vi "Event handler-Restart.vi"(11 "Queue in":refnum<queue>) -> (0 "error out":errorcluster)   [LabVIEW 2013]
uses:
  Queue/Message Queue/Typedefs/Message Cluster.ctl
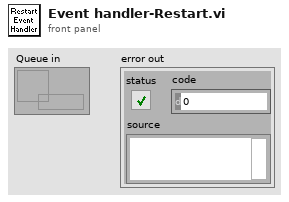
[diagram p1: front panel]
types:
  T1 = enum32{"Invalid", "Standard", "Closed", "Hidden", "Minimized", "Maximized"}
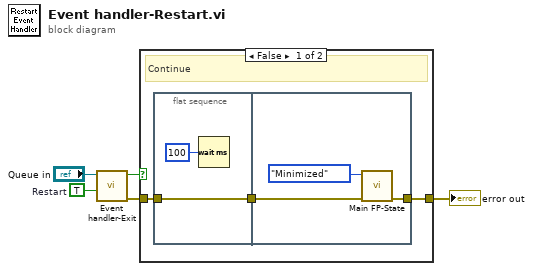
[diagram p0: block diagram]
diagram:
  w5 = TRUE  # Restart
  n1 = call "Event handler-Exit.vi"("Restart (F)"=w5, "UI queue"="Queue in") -> ("error out"=w1:errorcluster, "Cancelled"=w4:bool)  [unwired: 8 in]
  n2 = case shown="False" w4 {
    tunnel: [w8 w14] -> w2
    tunnel: w1 -> [w7 w14]
    frame False {
      # "Continue"
      n3 = flat-sequence {
        tunnel: [w10] -> w6
        tunnel: w7 -> [w10]
        tunnel: [w13] -> w8
        tunnel: w6 -> [w12]
        frame #0 {
          n4 = Wait (ms)(milliseconds to wait=u32 100) -> ()  [unwired: 1 out]
        }
        frame #1 {
          n5 = call "Main FP-State.vi"("error in (no error)"=w12, "Front Panel Window:State"=T1."Minimized") -> ("error out"=w13:errorcluster)  [unwired: 9 in]
        }
      }
    }
    frame True {
      # "Cancelled"
    }
  }
  "error out" <- w2
